vi "read_bin.vi"() -> ()   [LabVIEW 2020]
panel:
  out "size(s)":i32
  out "data":i16[](array[numeric])
  out "error out":errorcluster
  in  "file path (use dialog)":path
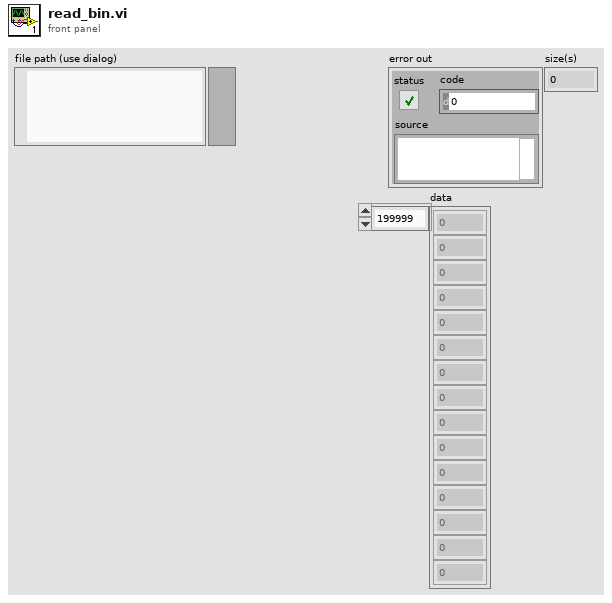
[diagram p1: front panel]
types:
  T1 = enum16{"big-endian, network order", "native, host order", "little-endian"}
  T2 = enum16{"open", "replace", "create", "open or create", "replace or create", "replace or create with confirmation"}
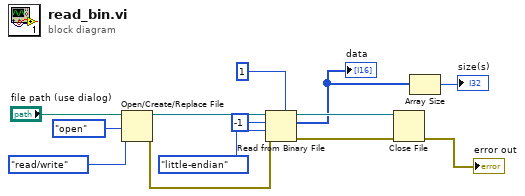
[diagram p0: block diagram]
diagram:
  n1 = Open/Create/Replace File(file path (use dialog)="file path (use dialog)", operation (0:open)=T2."open", access (0:read/write)=enum16{"read/write", "read-only", "write-only"}."read/write") -> (refnum out=w11:refnum<file>, error out=w10:errorcluster)  [unwired: 3 in, 1 out]
  n2 = Read from Binary File(5:i16 1 ("count (1)"), 8:w10, 9:T1."little-endian" ("byte order (0:big-endian, network order)"), 10:-1 ("count (1)"), 11:w11) -> (0:w9:errorcluster, 2:w2:i16[], 3:w12:refnum<file>)  [unwired: 1 in, 1 out]
  "data" <- w2
  n3 = Close File(refnum=w12, error in=w9) -> (error out=→"error out":errorcluster)  [unwired: 1 out]
  n4 = Array Size(array=w2) -> (size(s)=→"size(s)":i32)
